vi "Vision Processing.vi"(4 "error in (no error)":errorcluster, 5 "Camera Type":enum16{"206", "1011"}(ring)=enum."1011", 6 "Camera Name":string="Camera") -> ()   [LabVIEW 2012]
uses:
  Robot Global Data.vi
  <vilib>/vision/NI_Vision_Development_Module.lvlib
panel:
  out "Out Cirlcle Info":cluster{dbl, dbl}
  out "Circle Info":cluster{dbl, dbl, dbl}[](array[cluster])
  in  "Color Enabled":bool=TRUE
  in  "Range":cluster{"Lower value":sgl, "Upper value":sgl}={"Lower value"=151.52174, "Upper value"=255.0} {"Lower value" scale=0.0..255.0; "Upper value" scale=0.0..255.0}
  out "Out Target Info":cluster{"X":dbl, "Y":dbl, "Distance (ft)":dbl}
  in  "Enable Vision":bool=TRUE
  in  "View":bool
  out "Target Info":T1(array[cluster])
  in  "Area Size Limit %":dbl=0.5
  in  "Particle Count Limit":i32=8
  in  "Score Limits":T2={"Rect Coverage"=60.0, "X Edge Strength"=40.0, "Y Edge Strength"=60.0, "Center"=33.0, "Outer"=50.0}
  in  "View":bool
  out "Processed Image":T3(plugin-control)
  out "Original Image":T3(plugin-control)
  # "Instructions:\nProcessing the reflective tape that is illuminated by a ring light can be based\non color or light intensity.\nParticles within the image are scored by rectangle coverage, aspect ratio, and\nfor being hollow with a bold edge. A particle is considered a target if all scores\nare above the score limits. Particles can be annotated -- surrounded by\na rectangle and scores drawn to the left .\nTo control the number of particles being scored, use the count limit and the size\nlimit."
  # "To debug, Enable using the View button.\nFor color processing, you can click in the image to select the color for processing."
  # "Enable by clicking the View button.\nGreen scores are above the limit, orange are below. Inner/outer rect\nindicates all passed."
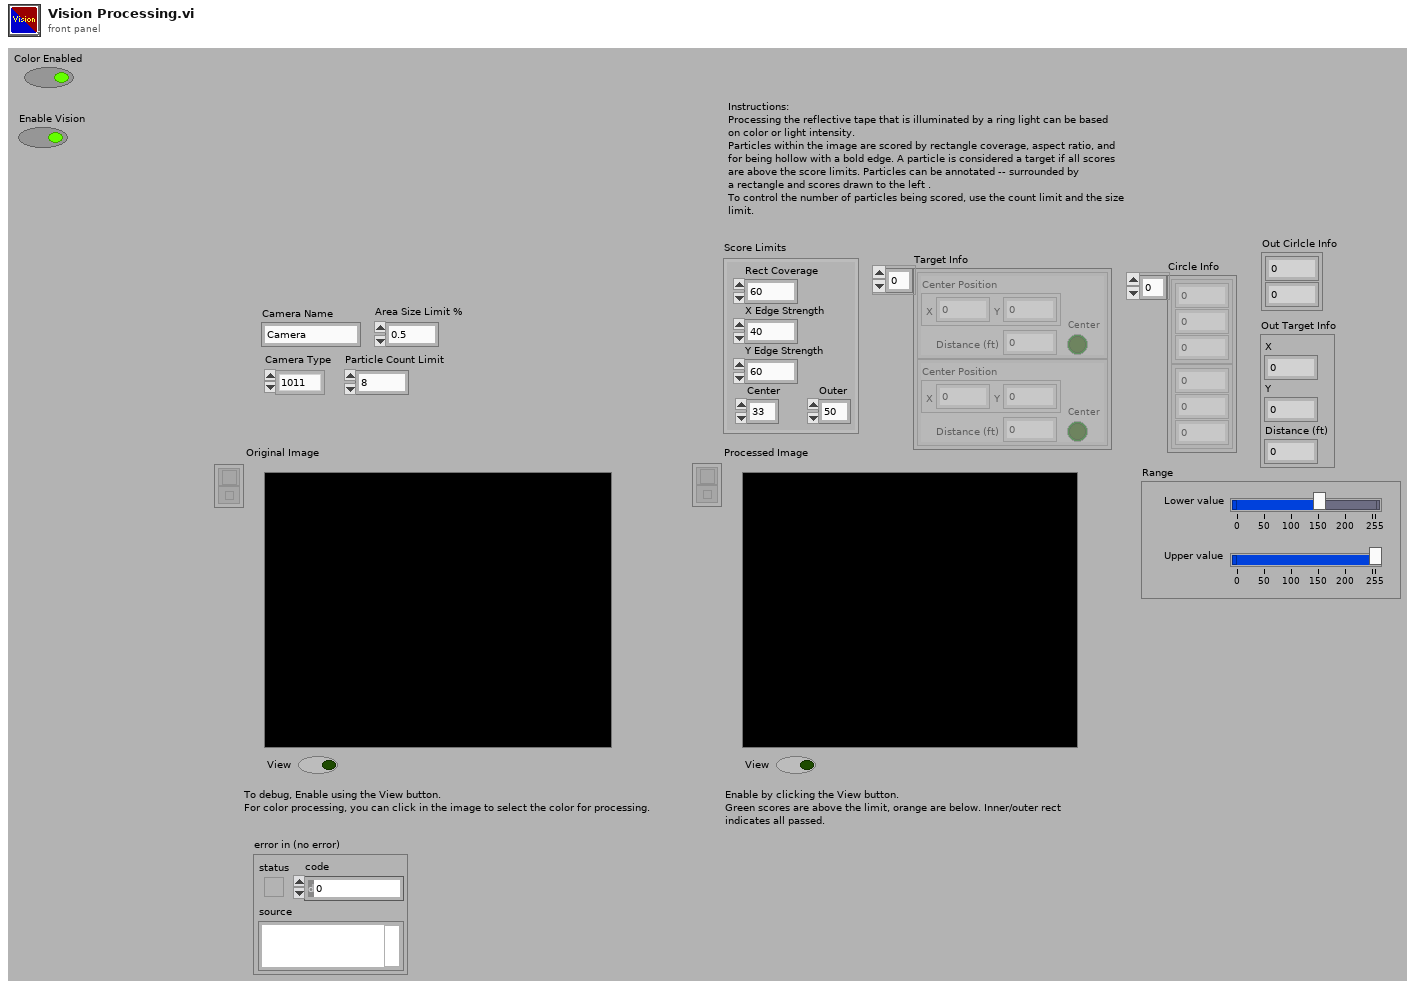
[diagram p1: front panel]
types:
  T1 = cluster{"Center Position":cluster{"X":dbl, "Y":dbl}, "Distance (ft)":dbl, "Center":bool}[]
  T2 = cluster{"Rect Coverage":dbl, "X Edge Strength":dbl, "Y Edge Strength":dbl, "Center":dbl, "Outer":dbl}
  T3 = typedef "IMAQ Image.ctl" = refnum<image>
  T4 = typedef "Image Type" = u32
  T5 = typedef "WPI_CameraDevRef.ctl" = cluster{"Camera Address":string, "CameraStatus":errorcluster, "Acquire Image Notifier":refnum<notifier>}
  T6 = cluster{"Position":cluster{"X":dbl, "Y":dbl}, "Distance (ft)":dbl, "Center":bool}[]
  T7 = typedef "WPI_CameraImageSize.ctl" = enum16{"640x480", "320x240", "160x120"}
  T8 = cluster{cluster{"Left":dbl, "Top":dbl, "Right":dbl, "Bottom":dbl}, "Scores":dbl[], cluster{"Long":dbl, "Short":dbl}}[]
  T9 = cluster{"Target Center (-1 to 1)":cluster{"X":dbl, "Y":dbl}, "Distance (ft)":dbl, "Center Target":bool}
  T10 = cluster{"Target Center (-1 to 1)":cluster{"X":dbl, "Y":dbl}, "Distance (ft)":dbl, "Center Target":bool}[]
  T11 = cluster{"Left":dbl, "Top":dbl, "Right":dbl, "Bottom":dbl}
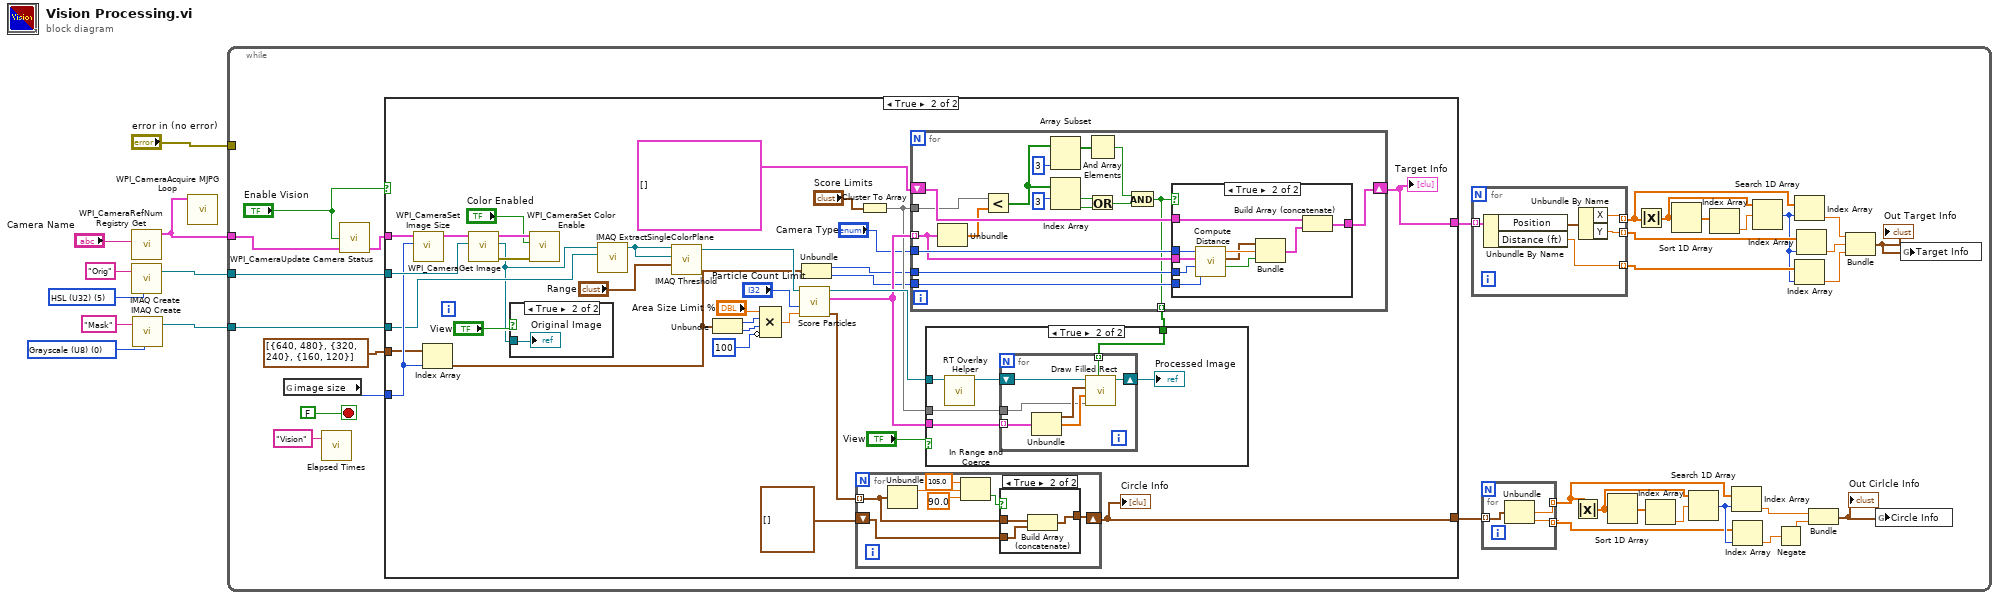
[diagram p0: block diagram]
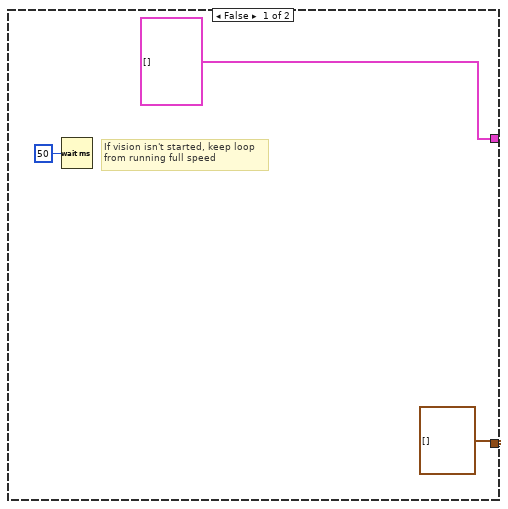
[diagram p2: hidden frame]
diagram:
  w3 = T4 0 items=["Grayscale (U8)", "Grayscale (I16)", "Grayscale (SGL)", "Complex (CSG)", "RGB (U32)", "HSL (U32)", "RGB (U64)", "Grayscale (U16)"] ("Image Type")
  w8 = T4 5 items=["Grayscale (U8)", "Grayscale (I16)", "Grayscale (SGL)", "Complex (CSG)", "RGB (U32)", "HSL (U32)", "RGB (U64)", "Grayscale (U16)"] ("Image Type")
  n1 = call <vilib>:"WPI_CameraRefNum Registry Get.vi"("refnum name"="Camera Name") -> ("CameraDevRef"=w5:T5)  [unwired: 9 in, 1 out]
  n2 = call "IMAQ Create"("Image Name"="Orig", "Image Type"=w8) -> ("New Image"=w7:T3)  [unwired: 2 in, 2 out]
  n3 = call "IMAQ Create"("Image Name"="Mask", "Image Type"=w3) -> ("New Image"=w1:T3)  [unwired: 2 in, 2 out]
  n4 = call <vilib>:"WPI_CameraAcquire MJPG Loop.vi"("CameraDevRef"=w5) -> ()  [unwired: 11 in]
  n5 = while {
    tunnel: w7 -> [w40]
    tunnel: w5 -> [w39]
    tunnel: "error in (no error)" -> [_]
    tunnel: w1 -> [w36]
    stop <- FALSE stop-if-true
    n6 = global read "Robot Global Data.vi" "image size"() -> (w37:T7)
    n7 = call "Elapsed Times.vi"("Call Name"="Vision") -> ()  [unwired: 2 in, 1 out]
    n8 = call <vilib>:"WPI_CameraUpdate Camera Status.vi"("CameraDevRef In"=w39, "Enable Vision"="Enable Vision") -> ("CameraDevRef Out"=w38:T5)  [unwired: 3 in]
    n9 = case shown="True" "Enable Vision" {
      tunnel: w40 -> [_ w82]
      tunnel: w38 -> [_ w78]
      tunnel: w37 -> [_ w75]
      tunnel: w36 -> [_ w71]
      tunnel: cluster{i32, i32}[] [{640, 480}, {320, 240}, {160, 120}] -> [_ w74]
      tunnel: [T6 [] w65] -> w32
      tunnel: [cluster{dbl, dbl, dbl}[] [] ("Circle Info 2") w53] -> w14
      frame False {
        # "If vision isn't started, keep loop\nfrom running full speed"
        n10 = Wait (ms)(milliseconds to wait=u32 50) -> ()  [unwired: 1 out]
      }
      frame True {
        n11 = call <vilib>:"WPI_CameraSet Image Size.vi"("Image Size"=w75, "CameraDevRef"=w78) -> ("CameraDevRef Out"=w79:T5)  [unwired: 8 in, 1 out]
        n12 = Index Array(array=w74, index=w75) -> (element=w66:cluster{i32, i32})
        n13 = call <vilib>:"WPI_CameraGet Image.vi"("Image"=w82, "CameraDevRef"=w79) -> ("error out"=w80:errorcluster, "Image Out"=w70:T3, "CameraDevRef Out"=w81:T5)  [unwired: 7 in]
        n14 = case shown="True" "View" {
          tunnel: w70 -> [_ w140]
          frame False {
          }
          frame True {
            "Original Image" <- w140
          }
        }
        n15 = call <vilib>:"WPI_CameraSet Color Enable.vi"("error in (no error)"=w80, "Color Enabled"="Color Enabled", "CameraDevRef"=w81) -> ()  [unwired: 7 in, 2 out]
        n16 = call "IMAQ ExtractSingleColorPlane"("Image Dst"=w71, "Image Src"=w70) -> ("Image Dst Out"=w63:T3)  [unwired: 8 in, 1 out]
        n17 = call "IMAQ Threshold"("Range"="Range", "Image Dst"=w63, "Image Src"=w63) -> ("Image Dst Out"=w76:T3)  [unwired: 3 in, 5 out]
        n18 = Unbundle(w66) -> (w59:i32, w58:i32)
        n19 = Compound Arithmetic op=MULTIPLY("Area Size Limit %", w59, w58, invert 100 ("length")) -> (w56:dbl)
        n20 = call "Score Particles.vi"("Area Size Limit"=w56, "Particle Count Limit"="Particle Count Limit", "Image Refnum in"=w76) -> ("Circle Info"=w55:cluster{dbl, dbl, dbl}[], "Scored Particle Info"=w85:T8, "Image Refnum out"=w87:T3)  [unwired: 6 in]
        n21 = Unbundle(w66) -> (w73:i32, w72:i32)
        n22 = for {
          tunnel: w55 -> [w90] mode=indexing
          shift-right: [w88] -> w53
          shift-left: cluster{dbl, dbl, dbl}[] [] ("Circle Info") -> [w89]
          n23 = Unbundle(w90) -> (w94:dbl)  [unwired: 2 out]
          n24 = In Range and Coerce(upper limit=105.0, x=w94, lower limit=90.0) -> (In Range?=w91:bool)  [unwired: 1 out]
          n25 = case shown="True" w91 {
            tunnel: w90 -> [_ w98]
            tunnel: w89 -> [w95 w97]
            tunnel: [w95 w96] -> w88
            frame False {
            }
            frame True {
              n26 = Build Array (concatenate)(w98, w97) -> (w96:cluster{dbl, dbl, dbl}[])
            }
          }
        }
        "Circle Info" <- w53
        n27 = Cluster To Array(cluster="Score Limits") -> (array=w83:dbl[])
        n28 = for {
          shift-right: [w114] -> w65
          shift-left: T6 [] -> [w115]
          tunnel: w73 -> [w113]
          tunnel: w85 -> [w108] mode=indexing
          tunnel: w83 -> [w110]
          tunnel: "Camera Type" -> [w112]
          tunnel: w72 -> [w109]
          tunnel: [w99] -> w67 mode=indexing
          n29 = Unbundle(w108) -> ("Scores"=w111:dbl[])  [unwired: 2 out]
          n30 = Less?(x=w110, y=w111) -> (x < y?=w100:bool[])
          n31 = Array Subset(array=w100, length=3) -> (w102:bool[])  [unwired: 1 in]
          n32 = Index Array(array=w100, index #1=3 ("length")) -> (element #1=w104:bool, element #2=w105:bool)  [unwired: 1 in]
          n33 = And Array Elements(Boolean array=w102) -> (logical AND=w107:bool)
          n34 = Or(x=w104, y=w105) -> (x .or. y?=w106:bool)
          n35 = And(x=w107, y=w106) -> (x .and. y?=w99:bool)
          n36 = case shown="True" w99 {
            tunnel: w115 -> [w116 w126]
            tunnel: [w116 w125] -> w114
            tunnel: w113 -> [_ w123]
            tunnel: w112 -> [_ w121]
            tunnel: w109 -> [_ w120]
            tunnel: w108 -> [_ w118]
            frame False {
            }
            frame True {
              n37 = call "Compute Distance.vi"("Y Image Resolution"=w120, "X Image Resolution"=w123, "Particle Scores"=w118, "Camera Type"=w121) -> ("Center Target"=w117:bool, "Target Center (-1 to 1)"=w119:cluster{"X":dbl, "Y":dbl}, "Distance (ft)"=w122:dbl)  [unwired: 5 in]
              n38 = Bundle("Target Center (-1 to 1)"=w119, "Distance (ft)"=w122, "Center Target"=w117) -> (w124:T9)  [unwired: 1 in]
              n39 = Build Array (concatenate)(w126, w124) -> (w125:T10)
            }
          }
        }
        "Target Info" <- w65
        n40 = case shown="True" "View" {
          tunnel: w87 -> [_ w129]
          tunnel: w85 -> [_ w131]
          tunnel: w83 -> [_ w130]
          tunnel: w67 -> [_ w127]
          frame False {
          }
          frame True {
            n41 = call "RT Overlay Helper.vi"("Refnum in"=w129) -> ("Refnum out"=w132:T3)  [unwired: 10 in]
            n42 = for {
              shift-right: [w138] -> w128
              shift-left: w132 -> [w139]
              tunnel: w131 -> [w135] mode=indexing
              tunnel: w130 -> [w134]
              tunnel: w127 -> [w133] mode=indexing
              n43 = Unbundle(w135) -> (w136:T11, "Scores"=w137:dbl[])  [unwired: 1 out]
              n44 = call "Draw Filled Rect.vi"("Limit Passed"=w133, "Limits"=w134, "Scores"=w137, "Bounding Box"=w136, "image in"=w139) -> ("image out"=w138:T3)  [unwired: 6 in]
            }
            "Processed Image" <- w128
          }
        }
      }
    }
    n45 = for {
      tunnel: w32 -> [w49] mode=indexing
      tunnel: [w47] -> w28 mode=indexing
      tunnel: [w46] -> w27 mode=indexing
      tunnel: [w45] -> w26 mode=indexing
      n46 = Unbundle By Name(w49) -> ("Position"=w48:cluster{"X":dbl, "Y":dbl}, "Distance (ft)"=w45:dbl)
      n47 = Unbundle By Name(w48) -> ("X"=w47:dbl, "Y"=w46:dbl)
    }
    n48 = for {
      tunnel: w14 -> [w44] mode=indexing
      tunnel: [w42] -> w18 mode=indexing
      tunnel: [w43] -> w19 mode=indexing
      n49 = Unbundle(w44) -> (w42:dbl, w43:dbl)  [unwired: 1 out]
    }
    n50 = Absolute Value(x=w18) -> (abs(x)=w16:dbl[])
    n51 = Sort 1D Array(array=w16) -> (sorted array=w15:dbl[])
    n52 = Absolute Value(x=w28) -> (abs(x)=w30:dbl[])
    n53 = Index Array(array=w15) -> (element=w17:dbl)  [unwired: 1 in]
    n54 = Sort 1D Array(array=w30) -> (sorted array=w31:dbl[])
    n55 = Search 1D Array(1D array=w16, element=w17) -> (index of element=w20:i32)  [unwired: 1 in]
    n56 = Index Array(array=w31) -> (element=w29:dbl)  [unwired: 1 in]
    n57 = Index Array(array=w18, index=w20) -> (element=w13:dbl)
    n58 = Index Array(array=w19, index=w20) -> (element=w11:dbl)
    n59 = Search 1D Array(1D array=w30, element=w29) -> (index of element=w25:i32)  [unwired: 1 in]
    n60 = Negate(x=w11) -> (-x=w10:dbl)
    n61 = Index Array(array=w28, index=w25) -> (element=w24:dbl)
    n62 = Index Array(array=w26, index=w25) -> (element=w22:dbl)
    n63 = Index Array(array=w27, index=w25) -> (element=w23:dbl)
    n64 = Bundle(w13, w10) -> (w12:cluster{dbl, dbl})  [unwired: 1 in]
    "Out Cirlcle Info" <- w12
    n65 = Bundle("X"=w24, "Y"=w23, "Distance (ft)"=w22) -> (w21:cluster{"X":dbl, "Y":dbl, "Distance (ft)":dbl})  [unwired: 1 in]
    "Out Target Info" <- w21
    n66 = global write "Robot Global Data.vi" "Circle Info"(w12) -> ()
    n67 = global write "Robot Global Data.vi" "Target Info"(w21) -> ()
  }
